vi "Disconnect.vi"(8 "error in (no error)":errorcluster, 11 "LNAX301 in":refnum<class "LNAX301.lvclass">) -> (0 "error out":errorcluster, 3 "LNAX301 out":refnum<class "LNAX301.lvclass">)   [LabVIEW 2017, in "LNAX301.lvclass"]
uses:
  LNAX301.lvclass
  Ctl/ITRI.ctl
  LNAX301.lvclass/LNAX301.ctl
  DLL/Modbus.dll
  <vilib>/NI/Modbus Library/API/Master/Modbus Master.lvclass
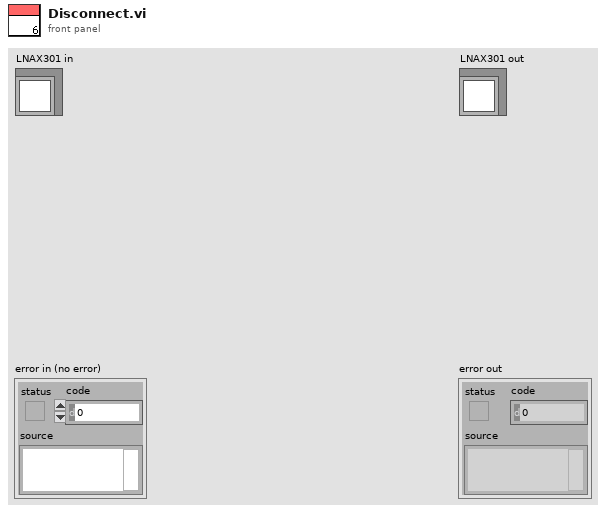
[diagram p1: front panel]
types:
  T1 = typedef "ITRI.ctl" = cluster{"amples in buffer":u16, "connect":bool, "CreateRtu":refnum<k24>, "SlaveID":u8, "Com port":string, "data":i16[]}
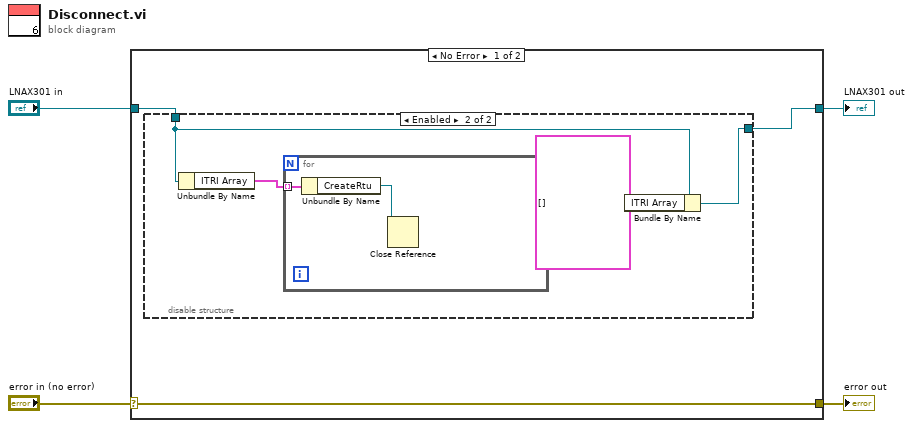
[diagram p0: block diagram]
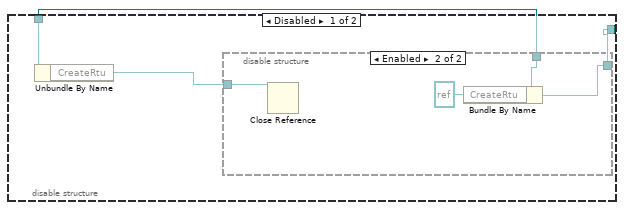
[diagram p2: hidden frame]
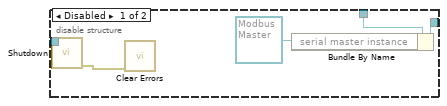
[diagram p3: hidden frame]
diagram:
  n1 = case shown="No Error" "error in (no error)" {
    selector: "error in (no error)" -> [w7 w27]
    tunnel: [w7 w27] -> w3
    tunnel: [w5 w26] -> w1
    tunnel: "LNAX301 in" -> [w6 w26]
    frame No Error {
      n2 = disable-structure shown="Enabled" {
        disable-tunnel: w6 -> [w9 w22]
        disable-tunnel: [w8 w20] -> w5
        frame Disabled {
          n3 = Unbundle By Name(w9) -> ("CreateRtu"=w10:refnum<k24>)
          n4 = disable-structure shown="Enabled" {
            disable-tunnel: w10 -> [w14 w19]
            disable-tunnel: w9 -> [w13 w18]
            disable-tunnel: [w12 w17] -> w8
            frame Disabled {
              n5 = call-dynamic "Shutdown.vi"("Modbus master in"=w14) -> ("error out"=w15:errorcluster)  [unwired: 10 in]
              n6 = call <vilib>:"Clear Errors.vi"("error in (no error)"=w15) -> ()  [unwired: 5 in, 2 out]
              n7 = Bundle By Name(cluster=w13, "serial master instance"=refnum<class "Modbus Master.lvclass"> refnum) -> (w12:refnum<class "LNAX301.lvclass">)
            }
            frame Enabled {
              n8 = Close Reference(reference=w19) -> ()  [unwired: 1 in, 1 out]
              n9 = Bundle By Name(cluster=w18, "CreateRtu"=refnum<k24> refnum) -> (w17:refnum<class "LNAX301.lvclass">)
            }
          }
        }
        frame Enabled {
          n10 = Unbundle By Name(w22) -> ("ITRI Array"=w23:T1[])
          n11 = for {
            tunnel: w23 -> [w25] mode=indexing
            n12 = Unbundle By Name(w25) -> ("CreateRtu"=w24:refnum<k24>)
            n13 = Close Reference(reference=w24) -> ()  [unwired: 1 in, 1 out]
          }
          n14 = Bundle By Name(cluster=w22, "ITRI Array"=T1[] []) -> (w20:refnum<class "LNAX301.lvclass">)
        }
      }
    }
    frame Error {
    }
  }
  "error out" <- w3
  "LNAX301 out" <- w1
